vi "Lock Data.vi"(6 "Wait for Confirmation Timeout [ms] (0=No Wait)":i32, 8 "error in (no error)":errorcluster, 9 "Datum Type":variant, 10 "Datum Name":string, 11 "IModel in":refnum<class "IModel.lvclass">) -> (0 "error out":errorcluster, 3 "IModel out":refnum<class "IModel.lvclass">)   [LabVIEW 2017, in "IModel.lvlib" / "IModel.lvclass"]
doc: "Publish a datum (value) to the mediator bus. Published data are observable by any actor with access to the mediated bus."
uses:
  IModel.lvclass
  C:/Git/mva-framework/Framework/IObserver/IObserver/IObserver.lvclass
  <vilib>/ActorFramework/Actor/Actor.lvclass/Actor.ctl
  <vilib>/ActorFramework/Message Enqueuer/Message Enqueuer.lvclass/Message Enqueuer.ctl
  IModel.lvclass/IModel.ctl
  Transport/QueueTransport/QueueTransport.lvclass/QueueTransport.ctl
  AbstractMessages/PreAddressedMsg/PreAddressedMsg.lvclass/PreAddressedMsg.ctl
  IMediator/IMediator Messages/Lock Publication Msg/Lock Publication Msg.lvclass/Lock Publication Msg.ctl
  <vilib>/ActorFramework/Actor/Read Self Enqueuer.vi
  <vilib>/ActorFramework/Message Enqueuer/Enqueue.vi
  AbstractMessages/PreAddressedMsg/Read Return Address.vi
  <vilib>/ActorFramework/Message Enqueuer/Init from Existing Queue.vi
  Transport/QueueTransport/QueueTransport.lvclass
  C:/Git/mva-framework/Framework/IMediator/ITransport/ITransport.lvclass
  IObserver/IObserver/IObserver.lvclass
  C:/Program Files (x86)/National Instruments/LabVIEW 2017/vi.lib/ActorFramework/Actor/Actor.lvclass
  IMediator/IMediator Messages/Lock Publication Msg/Lock Publication Msg.lvclass
  C:/Git/mva-framework/Framework/AbstractMessages/PreAddressedMsg/PreAddressedMsg.lvclass
  C:/Program Files (x86)/National Instruments/LabVIEW 2017/vi.lib/ActorFramework/Message/Message.lvclass
  <vilib>/Utility/error.llb/Error Cluster From Error Code.vi
  <vilib>/ActorFramework/Message Priority Queue/Priority Enqueue.vi
  IMediator/IPublicationPolicy/IPublicationPolicy.lvclass
  <vilib>/ActorFramework/Message Enqueuer/Message Enqueuer.lvclass
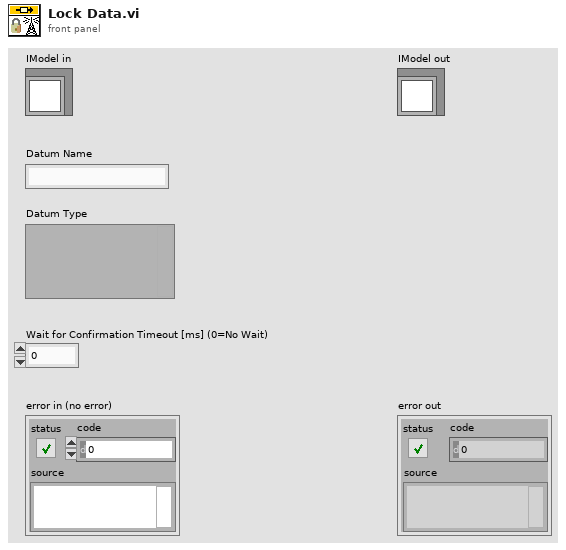
[diagram p1: front panel]
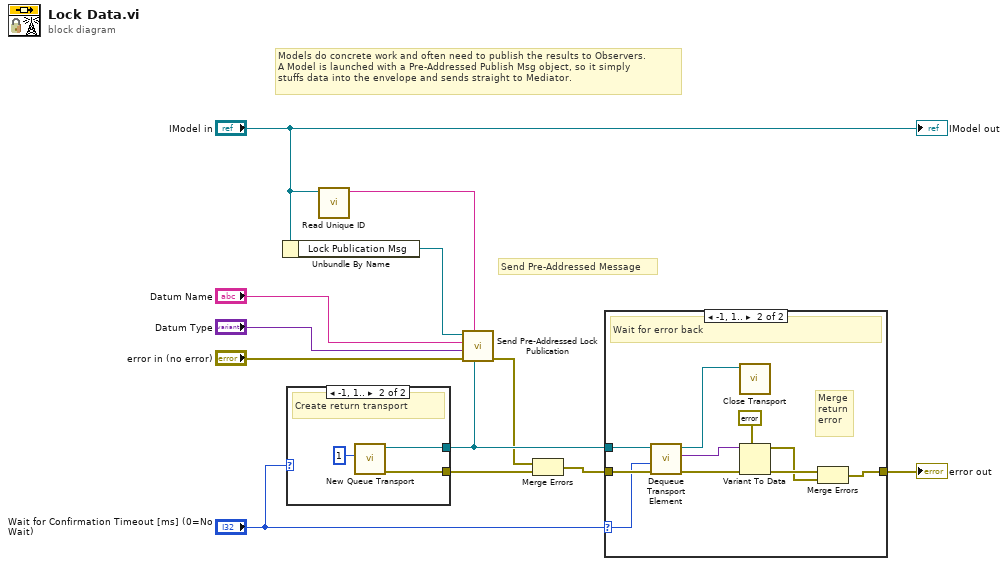
[diagram p0: block diagram]
diagram:
  # "Models do concrete work and often need to publish the results to Observers.\nA Model is launched with a Pre-Addressed Publish Msg object, so it simply\nstuffs data into the envelope and sends straight to Mediator."
  # "Send Pre-Addressed Message"
  n1 = Unbundle By Name("IModel in") -> ("Lock Publication Msg"=w12:refnum<class "Lock Publication Msg.lvclass">)
  n2 = case shown="-1, 1.." "Wait for Confirmation Timeout [ms] (0=No Wait)" {
    tunnel: [_ w14] -> w6
    tunnel: [_ w13] -> w3
    frame 0, Default {
      # "Do not handle return error"
    }
    frame -1, 1.. {
      # "Create return transport"
      n3 = call "New Queue Transport.vi"("Max Queue Size (-1)"=1) -> ("error out"=w13:errorcluster, "QueueTransport"=w14:refnum<class "QueueTransport.lvclass">)  [unwired: 9 in]
    }
  }
  n4 = call "Read Unique ID.vi"("IObserver In"="IModel in") -> ("Unique ID"=w8:string)  [unwired: 10 in]
  n5 = call "Send Pre-Addressed Lock Publication.vi"("Return Error Transport"=w6, "Publisher ID"=w8, "error in (no error)"="error in (no error)", "Data to Publish"="Datum Type", "Datum Name"="Datum Name", "Lock Publication Msg"=w12) -> ("error out"=w1:errorcluster)  [unwired: 5 in]
  n6 = Merge Errors(w1, w3) -> (w2:errorcluster)
  n7 = case shown="-1, 1.." "Wait for Confirmation Timeout [ms] (0=No Wait)" {
    selector: "Wait for Confirmation Timeout [ms] (0=No Wait)" -> [_ w24]
    tunnel: w6 -> [_ w26]
    tunnel: [w16 w18] -> w5
    tunnel: w2 -> [w16 w25]
    frame 0, Default {
      # "No wait"
    }
    frame -1, 1.. {
      # "Merge\nreturn\nerror"
      # "Wait for error back"
      n8 = call "Dequeue Transport Element.vi"("error in (no error)"=w25, "Timeout In ms (-1)"=w24, "QueueTransport in"=w26) -> ("error out"=w21:errorcluster, "Data"=w22:variant, "QueueTransport out"=w23:refnum<class "QueueTransport.lvclass">)  [unwired: 5 in, 1 out]
      n9 = call-dynamic "Close Transport.vi"("QueueTransport in"=w23) -> ()  [unwired: 10 in, 1 out]
      n10 = Variant To Data(error in=w21, type=errorcluster {"status"=FALSE, "code"=0, "source"=""} ("error constant"), Variant=w22) -> (data=w17:errorcluster, error out=w20:errorcluster)
      n11 = Merge Errors(w20, w17) -> (w18:errorcluster)
    }
  }
  "error out" <- w5
  "IModel out" <- "IModel in"
